vi "MFL_Manage_Monitor.vi"(3 "Lockin # (in)":i32, 4 "System Monitor Variables (in)":T3, 5 "Command (in)":T1 {"Osc 3 Freq" min=0.0 max=510000.0 format="%#_11g"; "Osc 2 Freq" min=0.0 max=510000.0 format="%#_11g"; "Osc 1 Freq" min=0.0 max=510000.0 format="%#_11g"; "Osc 0 Freq" min=0.0 max=510000.0 format="%#_11g"; "Demod Sample out 3"."Aux In 1 (V)" format="%#_5p"; "Demod Sample out 3"."Aux In 0 (V)" format="%#_5p"; "Demod Sample out 3"."X (Vrms)" format="%#_5p"; "Demod Sample out 3"."Y (Vrms)" format="%#_5p"; "Demod Sample out 3"."Osc Phase (rad)" format="%#.3g"; "Demod Sample out 2"."Aux In 1 (V)" format="%#_5p"; "Demod Sample out 2"."Aux In 0 (V)" format="%#_5p"; "Demod Sample out 2"."X (Vrms)" format="%#_5p"; "Demod Sample out 2"."Y (Vrms)" format="%#_5p"; "Demod Sample out 2"."Osc Phase (rad)" format="%#.3g"; "Demod Sample out 1"."Aux In 1 (V)" format="%#_5p"; "Demod Sample out 1"."Aux In 0 (V)" format="%#_5p"; "Demod Sample out 1"."X (Vrms)" format="%#_5p"; "Demod Sample out 1"."Y (Vrms)" format="%#_5p"; "Demod Sample out 1"."Osc Phase (rad)" format="%#.3g"; "Demod Sample out 0"."Aux In 1 (V)" format="%#_5p"; "Demod Sample out 0"."Aux In 0 (V)" format="%#_5p"; "Demod Sample out 0"."X (Vrms)" format="%#_5p"; "Demod Sample out 0"."Y (Vrms)" format="%#_5p"; "Demod Sample out 0"."Osc Phase (rad)" format="%#.3g"}, 6 "Global Status (in)":T1 {"Osc 3 Freq" min=0.0 max=510000.0 format="%#_11g"; "Osc 2 Freq" min=0.0 max=510000.0 format="%#_11g"; "Osc 1 Freq" min=0.0 max=510000.0 format="%#_11g"; "Osc 0 Freq" min=0.0 max=510000.0 format="%#_11g"; "Demod Sample out 3"."Aux In 1 (V)" format="%#_5p"; "Demod Sample out 3"."Aux In 0 (V)" format="%#_5p"; "Demod Sample out 3"."X (Vrms)" format="%#_5p"; "Demod Sample out 3"."Y (Vrms)" format="%#_5p"; "Demod Sample out 3"."Osc Phase (rad)" format="%#.3g"; "Demod Sample out 2"."Aux In 1 (V)" format="%#_5p"; "Demod Sample out 2"."Aux In 0 (V)" format="%#_5p"; "Demod Sample out 2"."X (Vrms)" format="%#_5p"; "Demod Sample out 2"."Y (Vrms)" format="%#_5p"; "Demod Sample out 2"."Osc Phase (rad)" format="%#.3g"; "Demod Sample out 1"."Aux In 1 (V)" format="%#_5p"; "Demod Sample out 1"."Aux In 0 (V)" format="%#_5p"; "Demod Sample out 1"."X (Vrms)" format="%#_5p"; "Demod Sample out 1"."Y (Vrms)" format="%#_5p"; "Demod Sample out 1"."Osc Phase (rad)" format="%#.3g"; "Demod Sample out 0"."Aux In 1 (V)" format="%#_5p"; "Demod Sample out 0"."Aux In 0 (V)" format="%#_5p"; "Demod Sample out 0"."X (Vrms)" format="%#_5p"; "Demod Sample out 0"."Y (Vrms)" format="%#_5p"; "Demod Sample out 0"."Osc Phase (rad)" format="%#.3g"}, 7 "queue (in)":refnum<queue>) -> (0 "Monitor (out)":T1 {"Osc 3 Freq" min=0.0 max=510000.0 format="%#_11g"; "Osc 2 Freq" min=0.0 max=510000.0 format="%#_11g"; "Osc 1 Freq" min=0.0 max=510000.0 format="%#_11g"; "Osc 0 Freq" min=0.0 max=510000.0 format="%#_11g"; "Demod Sample out 3"."Aux In 1 (V)" format="%#_5p"; "Demod Sample out 3"."Aux In 0 (V)" format="%#_5p"; "Demod Sample out 3"."X (Vrms)" format="%#_5p"; "Demod Sample out 3"."Y (Vrms)" format="%#_5p"; "Demod Sample out 3"."Osc Phase (rad)" format="%#.3g"; "Demod Sample out 2"."Aux In 1 (V)" format="%#_5p"; "Demod Sample out 2"."Aux In 0 (V)" format="%#_5p"; "Demod Sample out 2"."X (Vrms)" format="%#_5p"; "Demod Sample out 2"."Y (Vrms)" format="%#_5p"; "Demod Sample out 2"."Osc Phase (rad)" format="%#.3g"; "Demod Sample out 1"."Aux In 1 (V)" format="%#_5p"; "Demod Sample out 1"."Aux In 0 (V)" format="%#_5p"; "Demod Sample out 1"."X (Vrms)" format="%#_5p"; "Demod Sample out 1"."Y (Vrms)" format="%#_5p"; "Demod Sample out 1"."Osc Phase (rad)" format="%#.3g"; "Demod Sample out 0"."Aux In 1 (V)" format="%#_5p"; "Demod Sample out 0"."Aux In 0 (V)" format="%#_5p"; "Demod Sample out 0"."X (Vrms)" format="%#_5p"; "Demod Sample out 0"."Y (Vrms)" format="%#_5p"; "Demod Sample out 0"."Osc Phase (rad)" format="%#.3g"}, 1 "System Monitor Variables (out)":T3)   [LabVIEW 2019]
uses:
  Global/Global Variables/System Monitor Cluster.ctl
  zurich_lock_in/MFLIMonitor_Cluster.ctl
  Equipment/Zurich Instruments LabOne/Public/Data/ziTypeDemodSampleEx.ctl
  Instrument_Setup.vi
  Equipment/Zurich Instruments LabOne/Zurich Instruments LabOne.lvlib
panel:
  # "Oscillators"
  # "Output Amplitudes"
  # "Frequency (Hz)"
  # "Ampl (Vpk)"
  # "0"
  # "0"
  # "1"
  # "1"
  # "2"
  # "2"
  # "3"
  # "3"
  # "Oscillators"
  # "Output Amplitudes"
  # "Frequency (Hz)"
  # "Ampl (Vpk)"
  # "0"
  # "0"
  # "1"
  # "1"
  # "2"
  # "2"
  # "3"
  # "3"
  # "Oscillators"
  # "Output Amplitudes"
  # "Frequency (Hz)"
  # "Ampl (Vpk)"
  # "0"
  # "0"
  # "1"
  # "1"
  # "2"
  # "2"
  # "3"
  # "3"
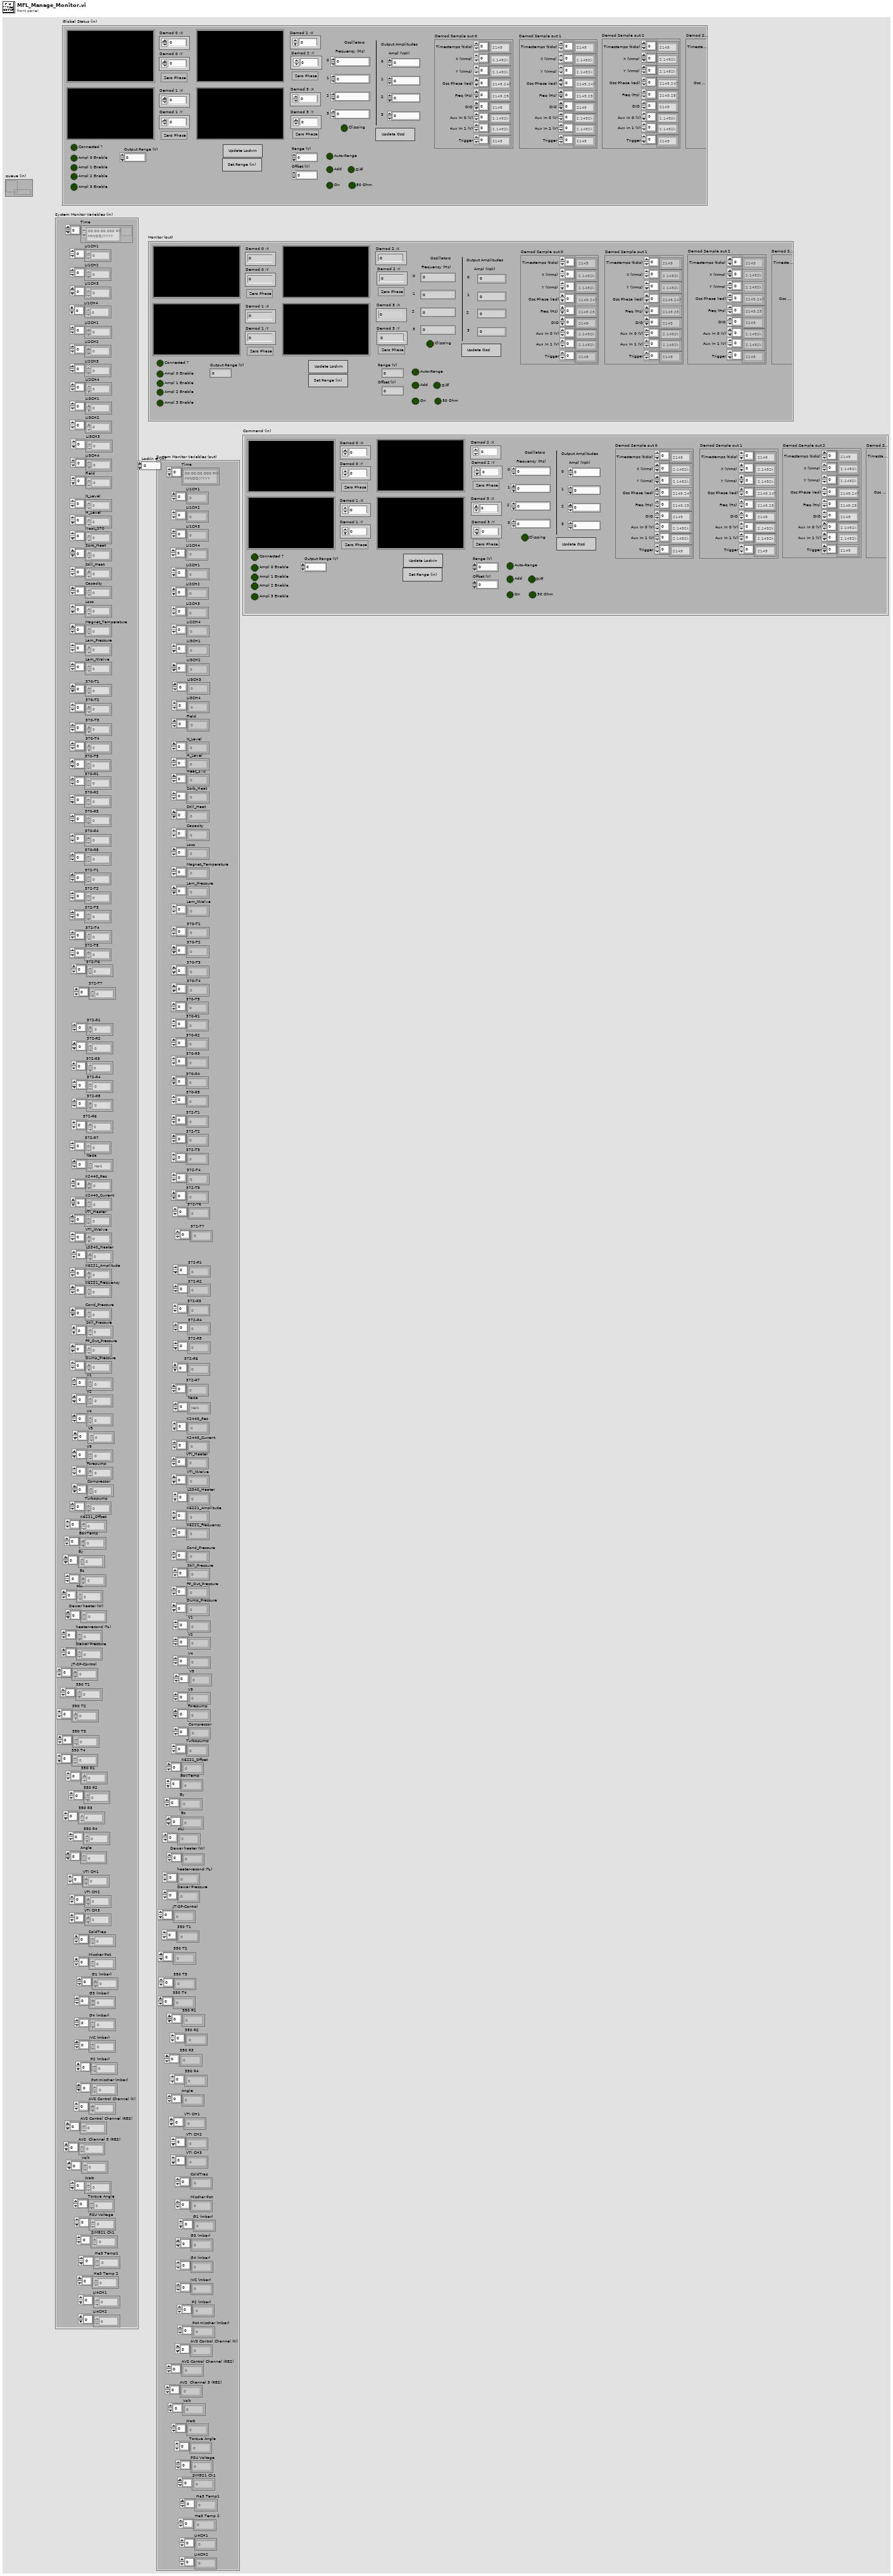
[diagram p1: front panel]
types:
  T1 = typedef "MFLIMonitor_Cluster.ctl" = cluster{"Demod 0":dbl[][], " Demod 1":dbl[][], "Demod 0 :X":dbl, "Demod 0 :Y ":dbl, "Demod 1 :X":dbl, "Demod 1 :Y ":dbl, " Demod 2":dbl[][], "Demod 3":dbl[][], "Demod 2 :X":dbl, "Demod 2 :Y ":dbl, "Demod 3 :X ":dbl, "Demod 3 :Y ":dbl, "Demod Sample out 0 ":T2, "Demod Sample out 1":T2, "Demod Sample out 2":T2, "Demod Sample out 3":T2, "Update Lock-In":bool, "Connected ?":bool, "Demod 0 Zero Phase":bool, "Demod 1 Zero Phase":bool, "Demod 2 Zero Phase":bool, "Demod 3 Zero Phase":bool, "Osc 0 Freq":dbl, "Osc 1 Freq":dbl, "Osc 2 Freq":dbl, "Osc 3 Freq":dbl, "Clipping":bool, "Range (V)":dbl, "Offset (V)":dbl, "Auto-Range":bool, "Add":bool, "Diff":bool, "On":bool, "50 Ohm":bool, "Ampl 0 Enable":bool, "Ampl 1 Enable":bool, "Ampl 2 Enable":bool, "Ampl 3 Enable":bool, "Ampl 0":dbl, "Ampl 1":dbl, "Ampl 2":dbl, "Ampl 3":dbl, "Update Osci":bool, "Output Range (V) ":dbl, "Set Range (in)":bool}
  T2 = typedef "Zurich Instruments LabOne.lvlib/ziTypeDemodSampleEx.ctl" = cluster{"Timestamps (ticks)":u64[], "X (Vrms)":dbl[], "Y (Vrms)":dbl[], "Osc Phase (rad)":dbl[], "Freq (Hz)":dbl[], "DIO":u32[], "Aux In 0 (V)":dbl[], "Aux In 1 (V)":dbl[], "Trigger":u32[]}
  T3 = typedef "System Monitor Cluster.ctl" = cluster{"Time":timestamp[], "LI1CH1":dbl[], "LI1CH2":dbl[], "LI2CH1":dbl[], "LI2CH2":dbl[], "LI3CH1":dbl[], "LI3CH2":dbl[], "Field":dbl[], "N_Level":dbl[], "H_Level":dbl[], "Heat_370":dbl[], "Sorb_Heat":dbl[], "Still_Heat":dbl[], "Capacity":dbl[], "Loss":dbl[], "Magnet_Temperature":dbl[], "Lam_Pressure":dbl[], "Lam_NValve":dbl[], "370-T1":dbl[], "370-T2":dbl[], "370-T3":dbl[], "370-T4":dbl[], "370-T5":dbl[], "370-R1":dbl[], "370-R2":dbl[], "370-R3":dbl[], "370-R4":dbl[], "370-R5":dbl[], "372-T1":dbl[], "372-T2":dbl[], "372-T3":dbl[], "372-T4":dbl[], "372-T5":dbl[], "372-T6":dbl[], "372-R1":dbl[], "372-R2":dbl[], "372-R3":dbl[], "372-R4":dbl[], "372-R5":dbl[], "372-R6":dbl[], "Nada":dbl[], "K2440_Res":dbl[], "K2440_Current":dbl[], "VTI_Heater":dbl[], "VTI_NValve":dbl[], "LS340_Heater":dbl[], "K6221_Amplitude":dbl[], "K6221_Frequency":dbl[], "Cond_Pressure":dbl[], "Still_Pressure":dbl[], "FP_Out_Pressure":dbl[], "Dump_Pressure":dbl[], "V1":dbl[], "V2":dbl[], "V4":dbl[], "V5":dbl[], "V9":dbl[], "Forepump":dbl[], "Compressor":dbl[], "K6221_Offset":dbl[], "BoxTemp":dbl[], "By":dbl[], "Bz":dbl[], "Phi":dbl[], "heater-recond (%)":dbl[], "Dewar Pressure ":dbl[], "JT-SP-Control":dbl[], "350 T1":dbl[], "350 T2":dbl[], "350 T3":dbl[], "350 T4":dbl[], "350 R1":dbl[], "350 R2":dbl[], "350 R3":dbl[], "350 R4":dbl[], "Angle":dbl[], "VTI CH1":dbl[], "VTI CH2":dbl[], "VTI CH3":dbl[], "ColdTrap":dbl[], "Mischer Pot":dbl[], "G1 (mbar)":dbl[], "G3 (mbar) ":dbl[], "G4 (mbar)":dbl[], "IVC (mbar)":dbl[], "P2 (mbar) ":dbl[], "Pot mischer (mbar)":dbl[], "AVS Control Channel (K)":dbl[], "AVS Control Channel (RES)":dbl[], "AVS  Channel 5 (RES) ":dbl[], "LI3CH3":dbl[], "LI3CH4":dbl[], "LI1CH3":dbl[], "LI1CH4":dbl[], "LI2CH3":dbl[], "LI2CH4":dbl[], "Volt":dbl[], "Watt":dbl[], "Torque Angle":dbl[], "Dewar heater (W)":dbl[], "PSU Voltage":dbl[], "Turbopump":dbl[], "372-R7":dbl[], "372-T7":dbl[], "SIM921 Ch1":dbl[], " He3 Temp1":dbl[], " He3 Temp 2":dbl[], "LI4CH1":dbl[], "LI4CH2":dbl[]}
  T4 = typedef "MFLIMonitor_Control_Cluster.ctl" = cluster{"Update Lock-In":bool, "Demod 0 Zero Phase":bool, "Demod 1 Zero Phase":bool, "Demod 2 Zero Phase":bool, "Demod 3 Zero Phase":bool, "Osc 0 Freq":dbl, "Osc 1 Freq":dbl, "Osc 2 Freq":dbl, "Osc 3 Freq":dbl, "Range (V)":dbl, "Offset (V)":dbl, "Ampl 0":dbl, "Ampl 1":dbl, "Ampl 2":dbl, "Ampl 3":dbl, "Update Osci":bool, "Output Range (V)":dbl, "Set Range (In)":bool}
  T5 = typedef "MFLIMonitor_Status_Cluster.ctl" = cluster{"Demod 0":dbl[][], " Demod 1":dbl[][], "Demod 0 :X":dbl, "Demod 0 :Y ":dbl, "Demod 1 :X":dbl, "Demod 1 :Y ":dbl, " Demod 2":dbl[][], "Demod 3":dbl[][], "Demod 2 :X":dbl, "Demod 2 :Y ":dbl, "Demod 3 :X ":dbl, "Demod 3 :Y ":dbl, "Demod Sample out 0 ":T2, "Demod Sample out 1":T2, "Demod Sample out 2":T2, "Demod Sample out 3":T2, "Connected ?":bool, "Clipping":bool, "Auto-Range":bool, "Add":bool, "Diff":bool, "On":bool, "50 Ohm":bool, "Ampl 0 Enable":bool, "Ampl 1 Enable":bool, "Ampl 2 Enable":bool, "Ampl 3 Enable":bool}
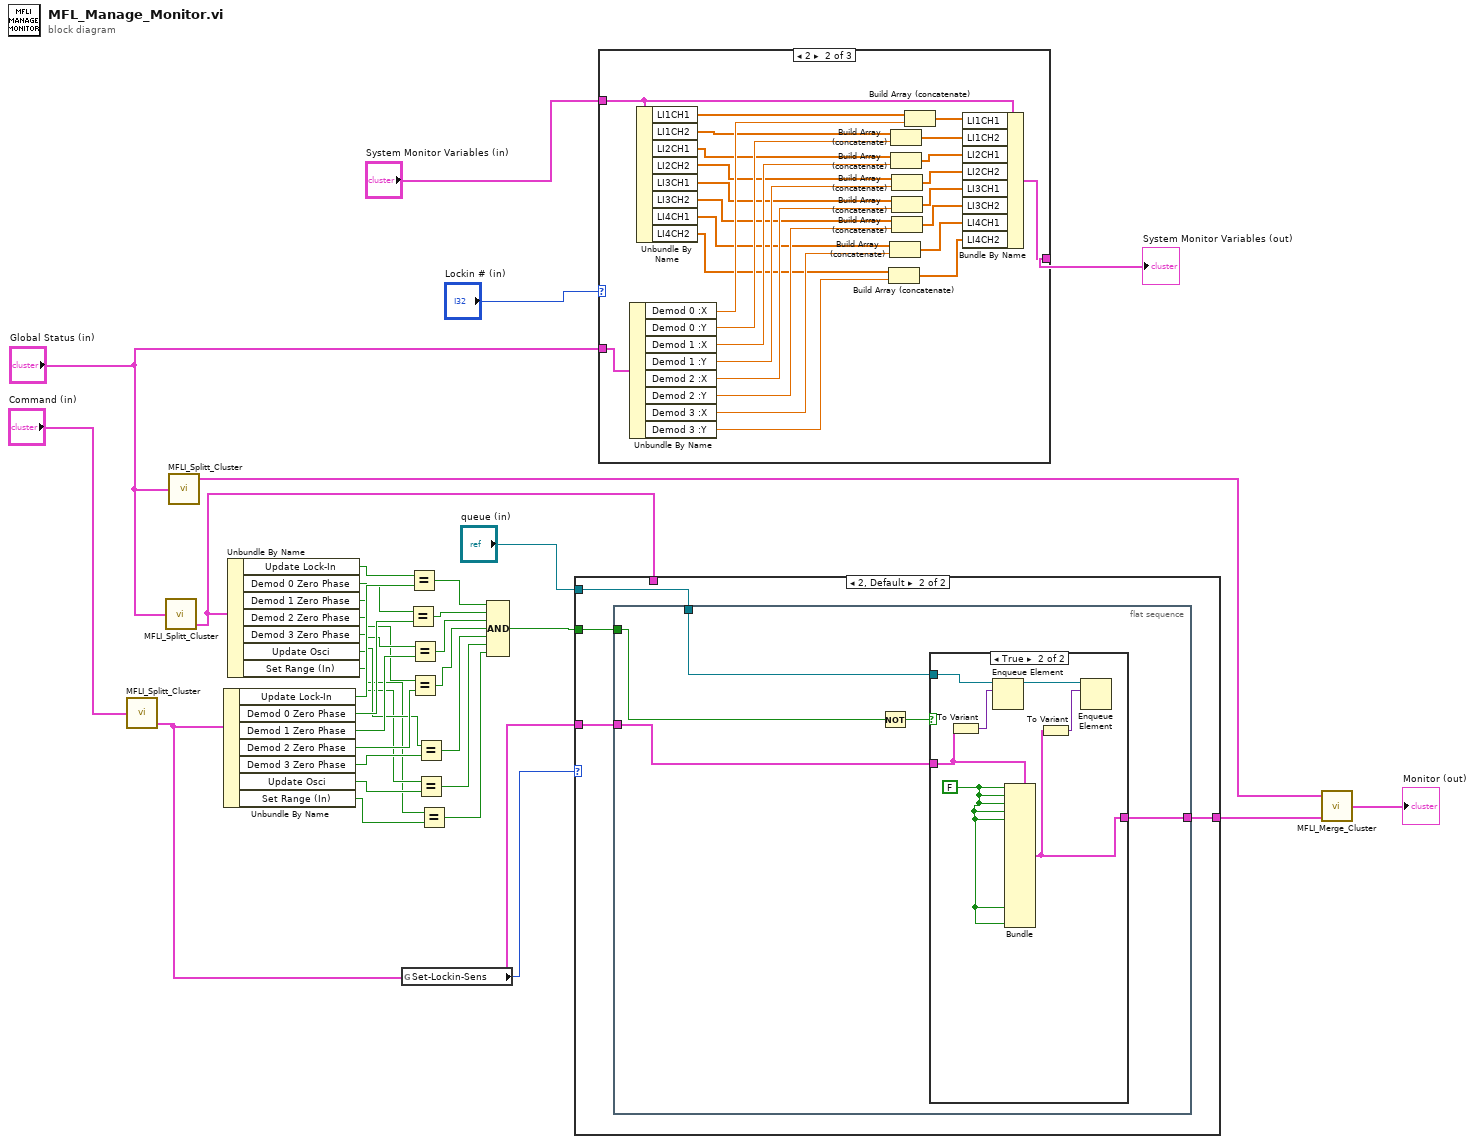
[diagram p0: block diagram]
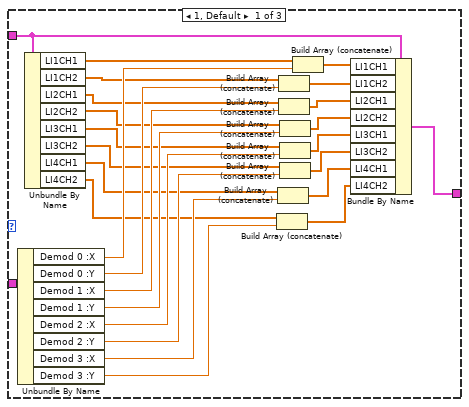
[diagram p4: hidden frame]
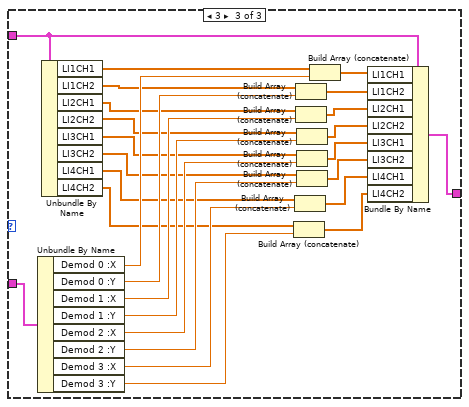
[diagram p5: hidden frame]
diagram:
  n1 = call "MFLI_Splitt_Cluster.vi"("MFL_Monitor"="Command (in)") -> ("MFL_Monitor Control"=w23:T4)  [unwired: 3 in, 1 out]
  n2 = call "MFLI_Splitt_Cluster.vi"("MFL_Monitor"="Global Status (in)") -> ("MFL_Monitor Control"=w25:T4)  [unwired: 3 in, 1 out]
  n3 = call "MFLI_Splitt_Cluster.vi"("MFL_Monitor"="Global Status (in)") -> ("MFL_Monitor Status"=w26:T5)  [unwired: 3 in, 1 out]
  n4 = Unbundle By Name(w23) -> ("Update Lock-In"=w21:bool, "Demod 0 Zero Phase"=w19:bool, "Demod 1 Zero Phase"=w17:bool, "Demod 2 Zero Phase"=w16:bool, "Demod 3 Zero Phase"=w13:bool, "Update Osci"=w11:bool, "Set Range (In)"=w2:bool)
  n5 = Unbundle By Name(w25) -> ("Update Lock-In"=w22:bool, "Demod 0 Zero Phase"=w20:bool, "Demod 1 Zero Phase"=w18:bool, "Demod 2 Zero Phase"=w15:bool, "Demod 3 Zero Phase"=w14:bool, "Update Osci"=w12:bool, "Set Range (In)"=w3:bool)
  n6 = global read "Instrument_Setup.vi" "Set-Lockin-Sens"() -> (w31:u16)
  n7 = Equal?(x=w20, y=w19) -> (x = y?=w9:bool)
  n8 = Equal?(x=w22, y=w21) -> (x = y?=w10:bool)
  n9 = Equal?(x=w18, y=w17) -> (x = y?=w8:bool)
  n10 = Equal?(x=w15, y=w16) -> (x = y?=w7:bool)
  n11 = Equal?(x=w14, y=w13) -> (x = y?=w6:bool)
  n12 = Equal?(x=w12, y=w11) -> (x = y?=w5:bool)
  n13 = Equal?(x=w3, y=w2) -> (x = y?=w1:bool)
  n14 = Compound Arithmetic op=AND(w10, w9, w8, w7, w6, w5, w1) -> (w4:bool)
  n15 = case shown="2, Default" w31 {
    tunnel: w4 -> [_ w39]
    tunnel: [w35 w38] -> w29
    tunnel: w23 -> [_ w37]
    tunnel: "queue (in)" -> [_ w36]
    tunnel: w25 -> [w35 _]
    frame 0, 1 {
    }
    frame 2, Default {
      n16 = flat-sequence {
        tunnel: w37 -> [w42]
        tunnel: [w43] -> w38
        tunnel: w39 -> [w41]
        tunnel: w36 -> [w40]
        frame #0 {
          n17 = Not(x=w41) -> (.not. x?=w44:bool)
          n18 = case shown="True" w44 {
            tunnel: w40 -> [_ w52]
            tunnel: w42 -> [w45 w50]
            tunnel: [w45 w47] -> w43
            frame False {
            }
            frame True {
              w46 = FALSE
              n19 = To Variant(anything=w50) -> (Variant=w51:variant)
              n20 = Enqueue Element(queue=w52, element=w51) -> (queue out=w49:refnum<queue>)  [unwired: 2 in, 2 out]
              n21 = Bundle(cluster=w50, "Update Lock-In"=w46, "Demod 0 Zero Phase"=w46, "Demod 1 Zero Phase"=w46, "Demod 2 Zero Phase"=w46, "Demod 3 Zero Phase"=w46, "Update Osci"=w46, "Set Range (In)"=w46) -> (w47:T4)  [unwired: 11 in]
              n22 = To Variant(anything=w47) -> (Variant=w48:variant)
              n23 = Enqueue Element(queue=w49, element=w48) -> ()  [unwired: 2 in, 3 out]
            }
          }
        }
      }
    }
  }
  n24 = case shown="2" "Lockin # (in)" {
    tunnel: "Global Status (in)" -> [w79 w80 w108]
    tunnel: "System Monitor Variables (in)" -> [w78 w83 w110]
    tunnel: [w71 w82 w109] -> w33
    frame 1, Default {
      n25 = Unbundle By Name(w79) -> ("Demod 0 :X"=w77:dbl, "Demod 0 :Y"=w73:dbl, "Demod 1 :X"=w69:dbl, "Demod 1 :Y"=w65:dbl, "Demod 2 :X"=w62:dbl, "Demod 2 :Y"=w59:dbl, "Demod 3 :X"=w56:dbl, "Demod 3 :Y"=w53:dbl)
      n26 = Unbundle By Name(w78) -> ("LI1CH1"=w76:dbl[], "LI1CH2"=w74:dbl[], "LI2CH1"=w70:dbl[], "LI2CH2"=w66:dbl[], "LI3CH1"=w63:dbl[], "LI3CH2"=w60:dbl[], "LI4CH1"=w57:dbl[], "LI4CH2"=w54:dbl[])
      n27 = Build Array (concatenate)(w54, w53) -> (w55:dbl[])
      n28 = Build Array (concatenate)(w57, w56) -> (w58:dbl[])
      n29 = Build Array (concatenate)(w74, w73) -> (w72:dbl[])
      n30 = Build Array (concatenate)(w70, w69) -> (w68:dbl[])
      n31 = Build Array (concatenate)(w66, w65) -> (w67:dbl[])
      n32 = Build Array (concatenate)(w63, w62) -> (w64:dbl[])
      n33 = Build Array (concatenate)(w60, w59) -> (w61:dbl[])
      n34 = Build Array (concatenate)(w76, w77) -> (w75:dbl[])
      n35 = Bundle By Name(cluster=w78, "LI1CH1"=w75, "LI1CH2"=w72, "LI2CH1"=w68, "LI2CH2"=w67, "LI3CH1"=w64, "LI3CH2"=w61, "LI4CH1"=w58, "LI4CH2"=w55) -> (w71:T3)
    }
    frame 2 {
      n36 = Unbundle By Name(w80) -> ("Demod 0 :X"=w106:dbl, "Demod 0 :Y"=w102:dbl, "Demod 1 :X"=w99:dbl, "Demod 1 :Y"=w95:dbl, "Demod 2 :X"=w92:dbl, "Demod 2 :Y"=w89:dbl, "Demod 3 :X"=w86:dbl, "Demod 3 :Y"=w81:dbl)
      n37 = Unbundle By Name(w83) -> ("LI1CH1"=w105:dbl[], "LI1CH2"=w103:dbl[], "LI2CH1"=w100:dbl[], "LI2CH2"=w96:dbl[], "LI3CH1"=w93:dbl[], "LI3CH2"=w90:dbl[], "LI4CH1"=w87:dbl[], "LI4CH2"=w84:dbl[])
      n38 = Build Array (concatenate)(w84, w81) -> (w85:dbl[])
      n39 = Build Array (concatenate)(w87, w86) -> (w88:dbl[])
      n40 = Build Array (concatenate)(w103, w102) -> (w101:dbl[])
      n41 = Build Array (concatenate)(w100, w99) -> (w98:dbl[])
      n42 = Build Array (concatenate)(w96, w95) -> (w97:dbl[])
      n43 = Build Array (concatenate)(w93, w92) -> (w94:dbl[])
      n44 = Build Array (concatenate)(w90, w89) -> (w91:dbl[])
      n45 = Build Array (concatenate)(w105, w106) -> (w104:dbl[])
      n46 = Bundle By Name(cluster=w83, "LI1CH1"=w104, "LI1CH2"=w101, "LI2CH1"=w98, "LI2CH2"=w97, "LI3CH1"=w94, "LI3CH2"=w91, "LI4CH1"=w88, "LI4CH2"=w85) -> (w82:T3)
    }
    frame 3 {
      n47 = Unbundle By Name(w108) -> ("Demod 0 :X"=w133:dbl, "Demod 0 :Y"=w129:dbl, "Demod 1 :X"=w126:dbl, "Demod 1 :Y"=w122:dbl, "Demod 2 :X"=w119:dbl, "Demod 2 :Y"=w116:dbl, "Demod 3 :X"=w113:dbl, "Demod 3 :Y"=w107:dbl)
      n48 = Unbundle By Name(w110) -> ("LI1CH1"=w132:dbl[], "LI1CH2"=w130:dbl[], "LI2CH1"=w127:dbl[], "LI2CH2"=w123:dbl[], "LI3CH1"=w120:dbl[], "LI3CH2"=w117:dbl[], "LI4CH1"=w114:dbl[], "LI4CH2"=w111:dbl[])
      n49 = Build Array (concatenate)(w111, w107) -> (w112:dbl[])
      n50 = Build Array (concatenate)(w114, w113) -> (w115:dbl[])
      n51 = Build Array (concatenate)(w130, w129) -> (w128:dbl[])
      n52 = Build Array (concatenate)(w127, w126) -> (w125:dbl[])
      n53 = Build Array (concatenate)(w123, w122) -> (w124:dbl[])
      n54 = Build Array (concatenate)(w120, w119) -> (w121:dbl[])
      n55 = Build Array (concatenate)(w117, w116) -> (w118:dbl[])
      n56 = Build Array (concatenate)(w132, w133) -> (w131:dbl[])
      n57 = Bundle By Name(cluster=w110, "LI1CH1"=w131, "LI1CH2"=w128, "LI2CH1"=w125, "LI2CH2"=w124, "LI3CH1"=w121, "LI3CH2"=w118, "LI4CH1"=w115, "LI4CH2"=w112) -> (w109:T3)
    }
  }
  "System Monitor Variables (out)" <- w33
  n58 = call "MFLI_Merge_Cluster.vi"("MFL_Monitor Control"=w29, "MFL_Monitor Status"=w26) -> ("MFL_Monitor"=→"Monitor (out)":T1)  [unwired: 3 in]
